vi "ScanListGlobal.vi"(7 "Action":T1, 11 "Set Value":string) -> (3 "Value Out":string)   [LabVIEW 2012]
uses:
  ScanListGlobalAction.ctl
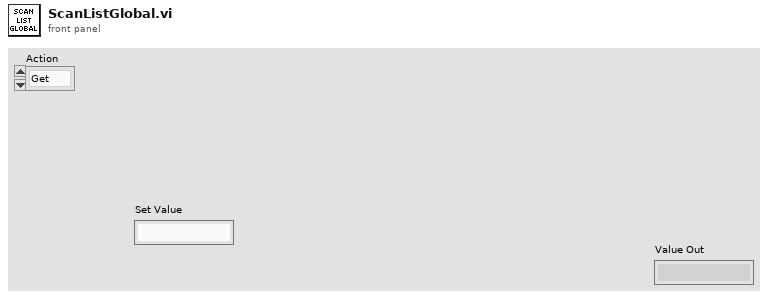
[diagram p1: front panel]
types:
  T1 = typedef "ScanListGlobalAction.ctl" = enum16{"Get", "Set", "Reset"}
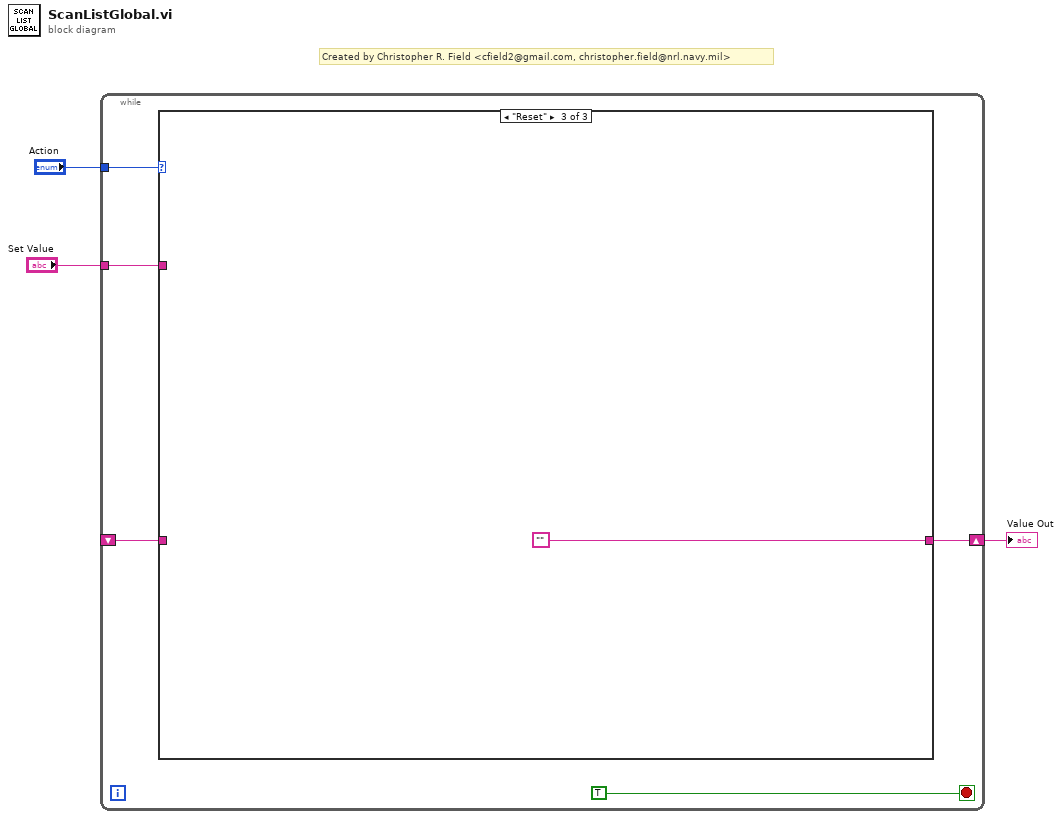
[diagram p0: block diagram]
diagram:
  # "Created by Christopher R. Field <cfield2@gmail.com, christopher.field@nrl.navy.mil>"
  n1 = while {
    tunnel: "Action" -> [w8]
    tunnel: "Set Value" -> [w6]
    shift-right: [w5] -> w1
    shift-left: _ -> [w4]
    stop <- TRUE stop-if-true
    n2 = case shown="\"Reset\"" w8 {
      tunnel: w6 -> [_ w10 _]
      tunnel: [w9 w10 ""] -> w5
      tunnel: w4 -> [w9 _ _]
      frame "Get", Default {
      }
      frame "Set" {
      }
      frame "Reset" {
      }
    }
  }
  "Value Out" <- w1
